vi "Server.vi"   [LabVIEW 2013]
uses:
  <vilib>/NXT/Block Support/NXT_MessageMailbox.ctl
  <vilib>/NXT/Dual Mode Library/Display/drawText.vi
types:
  T1 = typedef "LVHSConnector.ctl" = refnum<class "BrickReference.lvclass">
  T2 = typedef "NXT_MessageMailbox.ctl" = u8
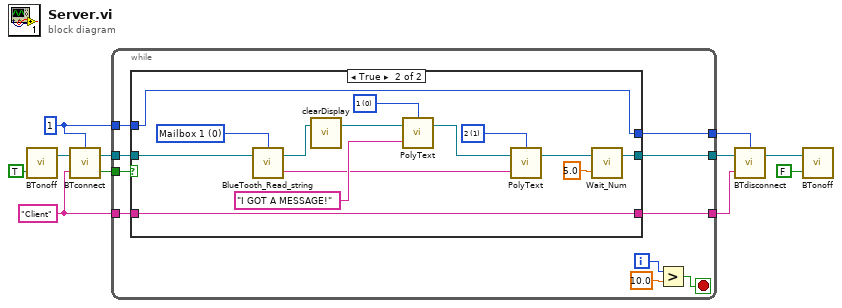
[diagram p0: block diagram]
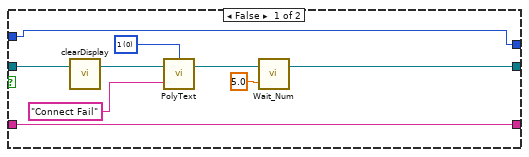
[diagram p2: hidden frame]
diagram:
  w2 = "Client" ("Partner Name")
  w7 = u8 1 ("Connection")
  n1 = call <vilib>:"BTonoff.vi"("On/Off"=TRUE) -> ("NXT/EV3"=w10:T1)  [unwired: 2 in, 1 out]
  n2 = call <vilib>:"BTconnect.vi"("Partner Name"=w2, "NXT/EV3"=w10, "Connection"=w7) -> ("Success"=w8:bool, "NXT/EV3"=w9:T1)
  n3 = while {
    tunnel: [w19] -> w5
    tunnel: w9 -> [w20]
    tunnel: w8 -> [w21]
    tunnel: w7 -> [w18]
    tunnel: [w17] -> w6
    tunnel: [w16] -> w3
    tunnel: w2 -> [w15]
    i -> [w13]
    stop <- w12 stop-if-true
    n4 = case shown="True" w21 {
      tunnel: w20 -> [w30 w44]
      tunnel: [w27 w33] -> w19
      tunnel: w18 -> [w22 w32]
      tunnel: [w22 w32] -> w17
      tunnel: [w23 w31] -> w16
      tunnel: w15 -> [w23 w31]
      frame False {
        w26 = i16 0 items=["1", "2", "3", "4", "5", "6", "7", "8", "9", "10", "11", "12"] ("Line")
        n5 = call <vilib>:"clearDisplay.vi"("NXT/EV3"=w30) -> ("NXT/EV3"=w29:T1)  [unwired: 3 in]
        n6 = call-poly <vilib>:"PolyText.vi"("Text"="Connect Fail", "NXT/EV3"=w29, "Line"=w26) -> ("NXT/EV3"=w28:T1)  [unwired: 1 in]
        n7 = call <vilib>:"Wait_Num.vi"("Time (1 sec)"=sgl 5.0, "NXT/EV3"=w28) -> ("NXT/EV3"=w27:T1)  [unwired: 2 in]
      }
      frame True {
        w34 = T2 0 items=["Mailbox 1", "Mailbox 2", "Mailbox 3", "Mailbox 4", "Mailbox 5", "Mailbox 6", "Mailbox 7", "Mailbox 8", "Mailbox 9", "Mailbox 10"] ("Mailbox")
        w35 = i16 1 items=["1", "2", "3", "4", "5", "6", "7", "8", "9", "10", "11", "12"] ("Line")
        w41 = i16 0 items=["1", "2", "3", "4", "5", "6", "7", "8", "9", "10", "11", "12"] ("Line")
        n8 = call <vilib>:"BlueTooth_Read_string.vi"("NXT/EV3"=w44, "Mailbox"=w34) -> ("Message"=w36:string, "NXT/EV3"=w43:T1)  [unwired: 1 in]
        n9 = call <vilib>:"clearDisplay.vi"("NXT/EV3"=w43) -> ("NXT/EV3"=w42:T1)  [unwired: 3 in]
        n10 = call-poly <vilib>:"PolyText.vi"("Text"="I GOT A MESSAGE!", "NXT/EV3"=w42, "Line"=w41) -> ("NXT/EV3"=w37:T1)  [unwired: 1 in]
        n11 = call-poly <vilib>:"PolyText.vi"("Text"=w36, "NXT/EV3"=w37, "Line"=w35) -> ("NXT/EV3"=w38:T1)  [unwired: 1 in]
        n12 = call <vilib>:"Wait_Num.vi"("Time (1 sec)"=sgl 5.0, "NXT/EV3"=w38) -> ("NXT/EV3"=w33:T1)  [unwired: 2 in]
      }
    }
    n13 = Greater?(x=w13, y=10.0) -> (0:w12:bool)
  }
  n14 = call <vilib>:"BTdisconnect.vi"("Partner Name"=w3, "NXT/EV3"=w5, "Connection"=w6) -> ("NXT/EV3"=w4:T1)  [unwired: 1 out]
  n15 = call <vilib>:"BTonoff.vi"("On/Off"=FALSE, "NXT/EV3"=w4) -> ()  [unwired: 1 in, 2 out]
